vi "DriveBegin.vi"(8 "error in (no error)":errorcluster) -> (0 "error out":errorcluster)   [LabVIEW 2020]
doc: "Begin for Drive\n\nInputs:\n -- Error in -- Error cluster -- propagated error input\n\nOutputs:\n -- Error out -- Error cluster -- progated error output"
uses:
  <vilib>/Rock Robotics/SystemInterfaces/DIO/FPGA_DIOChannel.ctl
  <vilib>/Rock Robotics/WPI/ThirdParty/Phoenix-LabVIEW/Motor Controller/Controls/CTRE_Phoenix_MotorControl_NeutralMode.ctl
  <vilib>/Rock Robotics/WPI/Counter/WPI_CounterDigitalInputToDigitalSource.vi
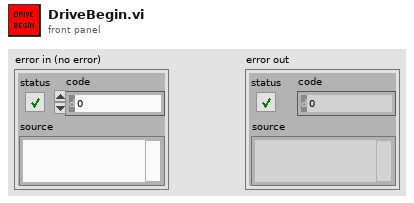
[diagram p1: front panel]
types:
  T1 = typedef "FPGA_DIOChannel.ctl" = enum8{"DIO 0", "DIO 1", "DIO 2", "DIO 3", "DIO 4", "DIO 5", "DIO 6", "DIO 7", "DIO 8", "DIO 9", "DIO MXP 0", "DIO MXP 1", "DIO MXP 2", "DIO MXP 3", "DIO MXP 4", "DIO MXP 5", "DIO MXP 6", "DIO MXP 7", "DIO MXP 8", "DIO MXP 9", "DIO MXP 10", "DIO MXP 11", "DIO MXP 12", "DIO MXP 13", "DIO MXP 14", "DIO MXP 15", "SPI Port CS1", "SPI Port CS2", "SPI Port CS3", "SPI Port MISO", "SPI Port MOSI", "Invalid"}
  T2 = typedef "CTRE_Phoenix_MotorControl_NeutralMode.ctl" = enum8{"EEPROMSetting", "Override to Coast", "Override to Brake"}
  T3 = typedef "WPI_MotorControlDeviceRef.ctl" = cluster{"DeviceStatus":errorcluster, "Type":T4, "PWM":cluster{"PWM Channel":T5, "DeadBand":T6}, "CAN":cluster{"Device Number":u8, "SetOutput VI Ref":variant, "GetOutput VI Ref":variant, "Enable VI Ref":variant, "Disable VI Ref":variant, "Data":variant}, "Invert":bool, "DIO PWM":cluster{"PWM \"Enable\" Channel":T5, "DIOChannel":T1, "PWM Rate":dbl}}
  T4 = typedef "WPI_MotorControlType.ctl" = enum16{"PWM", "CAN", "DIO PWM"}
  T5 = typedef "FPGA_DIOPWMChannel.ctl" = enum8{"PWM 0", "PWM 1", "PWM 2", "PWM 3", "PWM 4", "PWM 5", "PWM 6", "PWM 7", "PWM 8", "PWM 9", "PWM MXP 0", "PWM MXP 1", "PWM MXP 2", "PWM MXP 3", "PWM MXP 4", "PWM MXP 5", "PWM MXP 6", "PWM MXP 7", "PWM MXP 8", "PWM MXP 9", "Invalid"}
  T6 = typedef "WPI_PWMDeadband.ctl" = cluster{"Name":string, "maxPositivePwm":i32, "minPositivePwm":i32, "centerPwm":i32, "maxNegativePwm":i32, "minNegativePwm":i32, "angularRange":u16}
  T7 = typedef "WPI_DigitalInputDevRef.ctl" = cluster{"DevStatus":errorcluster, "DIO Channel":T1}
  T8 = typedef "FPGA_CounterEncoderSourceConvertionLVSourceType.ctl" = cluster{"DevStatus":errorcluster, "AnalogTriggerMode?":bool, "DigitalMode":cluster{"DIO Channel":T9}, "AnalogTriggerMode":cluster{"AnalogTriggerIndex":T10, "OutputType":T11}}
  T9 = typedef "FPGA_DIODigitalSourceChannel.ctl" = enum8{"DIO 0", "DIO 1", "DIO 2", "DIO 3", "DIO 4", "DIO 5", "DIO 6", "DIO 7", "DIO 8", "DIO 9", "DIO MXP 0", "DIO MXP 1", "DIO MXP 2", "DIO MXP 3", "DIO MXP 4", "DIO MXP 5", "DIO MXP 6", "DIO MXP 7", "DIO MXP 8", "DIO MXP 9", "DIO MXP 10", "DIO MXP 11", "DIO MXP 12", "DIO MXP 13", "DIO MXP 14", "DIO MXP 15", "SPI Port CS1", "SPI Port CS2", "SPI Port CS3", "SPI Port MISO", "SPI Port MOSI", "Disabled"}
  T10 = typedef "FPGA_AnalogTriggerIndex.ctl" = enum8{"Trig 0", "Trig 1", "Trig 2", "Trig 3", "Trig 4", "Trig 5", "Trig 6", "Trig 7", "Invalid"}
  T11 = typedef "FPGA_AnalogTriggerOutType.ctl" = enum16{"InWindow", "TriggerState", "Rising", "Falling"}
  T12 = typedef "ADIS16470 Device Reference.ctl" = cluster{"DevStatus":errorcluster, "Hardware Config":T13, "Calibration Complete":refnum<notifier>, "Status Reference":refnum<data-value>, "Data Reference":refnum<data-value>, "Sychronous Process VI":T16, "Cmd FIFO":refnum<k33>, "Source":T8, "Data FIFO":refnum<k33>, "Calibration Time (ms)":u32, "Data Reference":refnum<data-value>}
  T13 = typedef "ADIS16470 Hardware Configuration.ctl" = cluster{"SPI Clock Rate (Hz)":dbl, "IMU SPI Mode (3)":T14, "IMU Reset Pin":T1, "IMU SPI Bus":T15, "IMU Data Ready Pin":T1, "Stall Config":cluster{"Pow2BytesPerRead":u8, "StallTicks":u16, "CsToSclkTicks":u8}}
  T14 = typedef "WPI_SPIMode.ctl" = enum16{"Mode 0 (Clk Idle Low,Sample on Leading)", "Mode 1 (Clk Idle Low,Sample on Trailing)", "Mode 2 (Clk Idle High,Sample on Leading)", "Mode 3 (Clk Idle High,Sample on Trailing)"}
  T15 = typedef "spi_bus.ctl" = enum16{"SPI On-Board, CS0", "SPI On-Board, CS1", "SPI On-Board, CS2", "SPI On-Board, CS3", "SPI MXP", "Invalid"}
  T16 = typedef "ADIS16470 Process.ctl" = refnum<vi>
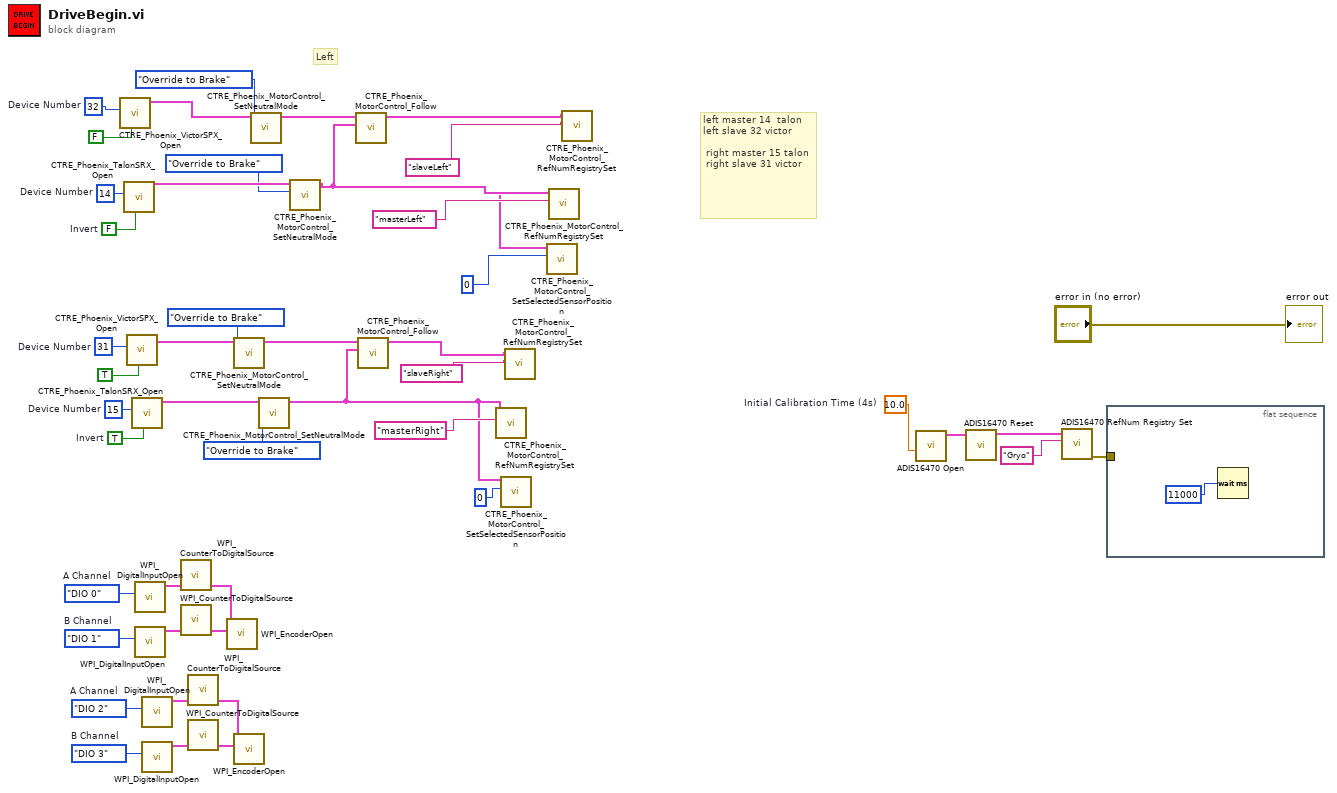
[diagram p0: block diagram]
diagram:
  w4 = FPGA_DIOChannel."DIO 3"  # B Channel
  w3 = FPGA_DIOChannel."DIO 2"  # A Channel
  w10 = FPGA_DIOChannel."DIO 1"  # B Channel
  w9 = FPGA_DIOChannel."DIO 0"  # A Channel
  w15 = u8 31  # Device Number
  w18 = u8 32  # Device Number
  w39 = 10.0  # Initial Calibration Time (4s)
  w41 = FALSE  # Invert
  w42 = TRUE  # Invert
  w44 = u8 15  # Device Number
  w43 = u8 14  # Device Number
  # "Left"
  # "left master 14  talon\nleft slave 32 victor\n\n\tright master 15 talon\n\tright slave 31 victor"
  n1 = call <vilib>:"CTRE_Phoenix_VictorSPX_Open.vi"("Invert"=FALSE, "Device Number"=w18) -> ("PhoenixMotorControlDevRef"=w13:T3)  [unwired: 8 in, 1 out]
  n2 = call <vilib>:"CTRE_Phoenix_TalonSRX_Open.vi"("Invert"=w41, "Device Number"=w43) -> ("PhoenixMotorControlDevRef"=w34:T3)  [unwired: 8 in, 1 out]
  n3 = call <vilib>:"CTRE_Phoenix_VictorSPX_Open.vi"("Invert"=TRUE, "Device Number"=w15) -> ("PhoenixMotorControlDevRef"=w16:T3)  [unwired: 8 in, 1 out]
  n4 = call <vilib>:"CTRE_Phoenix_TalonSRX_Open.vi"("Invert"=w42, "Device Number"=w44) -> ("PhoenixMotorControlDevRef"=w36:T3)  [unwired: 8 in, 1 out]
  n5 = call <vilib>:"WPI_DigitalInputOpen.vi"("DIO Channel"=w9) -> ("DigitalInputDevRef"=w7:T7)  [unwired: 1 in, 9 out]
  n6 = call <vilib>:"WPI_DigitalInputOpen.vi"("DIO Channel"=w10) -> ("DigitalInputDevRef"=w8:T7)  [unwired: 1 in, 9 out]
  n7 = call <vilib>:"WPI_DigitalInputOpen.vi"("DIO Channel"=w3) -> ("DigitalInputDevRef"=w1:T7)  [unwired: 1 in, 9 out]
  n8 = call <vilib>:"WPI_DigitalInputOpen.vi"("DIO Channel"=w4) -> ("DigitalInputDevRef"=w2:T7)  [unwired: 1 in, 9 out]
  n9 = call-poly <vilib>:"WPI_CounterToDigitalSource.vi"("DigitalInputDevRef"=w7) -> ("Digital Source"=w11:T8)  [unwired: 6 out]
  n10 = call-poly <vilib>:"WPI_CounterToDigitalSource.vi"("DigitalInputDevRef"=w8) -> ("Digital Source"=w12:T8)  [unwired: 6 out]
  n11 = call-poly <vilib>:"WPI_CounterToDigitalSource.vi"("DigitalInputDevRef"=w1) -> ("Digital Source"=w5:T8)  [unwired: 6 out]
  n12 = call-poly <vilib>:"WPI_CounterToDigitalSource.vi"("DigitalInputDevRef"=w2) -> ("Digital Source"=w6:T8)  [unwired: 6 out]
  n13 = call <vilib>:"WPI_EncoderOpen.vi"("BSource"=w12, "ASource"=w11) -> ()  [unwired: 8 in, 2 out]
  n14 = call <vilib>:"CTRE_Phoenix_MotorControl_SetNeutralMode.vi"("Motor Control Neutral Mode"=CTRE_Phoenix_MotorControl_NeutralMode."Override to Brake", "PhoenixMotorControlDevRef"=w16) -> ("PhoenixMotorControlDevRef"=w26:T3)  [unwired: 8 in, 1 out]
  n15 = call <vilib>:"WPI_EncoderOpen.vi"("BSource"=w6, "ASource"=w5) -> ()  [unwired: 8 in, 2 out]
  n16 = call <vilib>:"CTRE_Phoenix_MotorControl_SetNeutralMode.vi"("Motor Control Neutral Mode"=CTRE_Phoenix_MotorControl_NeutralMode."Override to Brake", "PhoenixMotorControlDevRef"=w13) -> ("PhoenixMotorControlDevRef"=w30:T3)  [unwired: 8 in, 1 out]
  n17 = call <vilib>:"CTRE_Phoenix_MotorControl_SetNeutralMode.vi"("Motor Control Neutral Mode"=CTRE_Phoenix_MotorControl_NeutralMode."Override to Brake", "PhoenixMotorControlDevRef"=w36) -> ("PhoenixMotorControlDevRef"=w19:T3)  [unwired: 8 in, 1 out]
  n18 = call <vilib>:"CTRE_Phoenix_MotorControl_SetNeutralMode.vi"("Motor Control Neutral Mode"=CTRE_Phoenix_MotorControl_NeutralMode."Override to Brake", "PhoenixMotorControlDevRef"=w34) -> ("PhoenixMotorControlDevRef"=w29:T3)  [unwired: 8 in, 1 out]
  n19 = call <vilib>:"CTRE_Phoenix_MotorControl_Follow.vi"("Master Controller to Follow"=w29, "PhoenixMotorControlDevRef"=w30) -> ("PhoenixMotorControlDevRef"=w28:T3)  [unwired: 8 in, 1 out]
  n20 = call <vilib>:"CTRE_Phoenix_MotorControl_Follow.vi"("Master Controller to Follow"=w19, "PhoenixMotorControlDevRef"=w26) -> ("PhoenixMotorControlDevRef"=w25:T3)  [unwired: 8 in, 1 out]
  n21 = call <vilib>:"CTRE_Phoenix_MotorControl_RefNumRegistrySet.vi"("refnum name"="masterRight", "PhoenixMotorControlDevRef"=w19) -> ()  [unwired: 8 in, 2 out]
  n22 = call <vilib>:"CTRE_Phoenix_MotorControl_SetSelectedSensorPosition.vi"("New Sensor Position"=0, "PhoenixMotorControlDevRef"=w19) -> ()  [unwired: 8 in, 2 out]
  n23 = call <vilib>:"CTRE_Phoenix_MotorControl_RefNumRegistrySet.vi"("refnum name"="slaveRight", "PhoenixMotorControlDevRef"=w25) -> ()  [unwired: 8 in, 2 out]
  n24 = call <vilib>:"CTRE_Phoenix_MotorControl_RefNumRegistrySet.vi"("refnum name"="masterLeft", "PhoenixMotorControlDevRef"=w29) -> ("PhoenixMotorControlDevRef"=w20:T3)  [unwired: 8 in, 1 out]
  n25 = call <vilib>:"CTRE_Phoenix_MotorControl_SetSelectedSensorPosition.vi"("New Sensor Position"=0, "PhoenixMotorControlDevRef"=w20) -> ()  [unwired: 8 in, 2 out]
  n26 = call <vilib>:"CTRE_Phoenix_MotorControl_RefNumRegistrySet.vi"("refnum name"="slaveLeft", "PhoenixMotorControlDevRef"=w28) -> ()  [unwired: 8 in, 2 out]
  n27 = call <vilib>:"ADIS16470 Open.vi"("Initial Calibration Time (4s)"=w39) -> ("ADIS16470DevRef"=w38:T12)  [unwired: 9 in, 1 out]
  n28 = call <vilib>:"ADIS16470 Reset.vi"("ADIS16470DevRef"=w38) -> ("ADIS16470DevRef"=w37:T12)  [unwired: 9 in, 1 out]
  n29 = call <vilib>:"ADIS16470 RefNum Registry Set.vi"("refnum name"="Gryo", "ADIS16470DevRef in"=w37) -> ("error out"=w32:errorcluster)  [unwired: 8 in, 1 out]
  n30 = flat-sequence {
    tunnel: w32 -> [_]
    frame #0 {
      n31 = Wait (ms)(milliseconds to wait=u32 11000) -> ()  [unwired: 1 out]
    }
  }
  "error out" <- "error in (no error)"
